vi "HeaderAction.vi"(0 "GenData en entrée":refnum<class "Tools.lvclass"> caption="DNL_LabVIEW Object in", 11 "error in (no error)":errorcluster caption="entrée d'erreur (pas d'erreur)") -> (4 "GenData en sortie":refnum<class "Tools.lvclass"> caption="DNL_LabVIEW Object out", 6 "DataNames":string[](array[string]), 8 "Instr Name":string, 10 "HeaderString":string, 13 "ArrDisplayNames":string[](array[string]), 14 "DisplayNames":string[](array[string]), 15 "error out":errorcluster caption="sortie d'erreur")   [LabVIEW 2019, in "Tools.lvclass"]
uses:
  Tools.lvclass
  C:/Programmes Labview/LabScanV1A/DevicesClass/BaseDevice/BaseDevice.lvclass
  Tools.lvclass/Tools.ctl
  BaseDevice/BaseDevice.lvclass
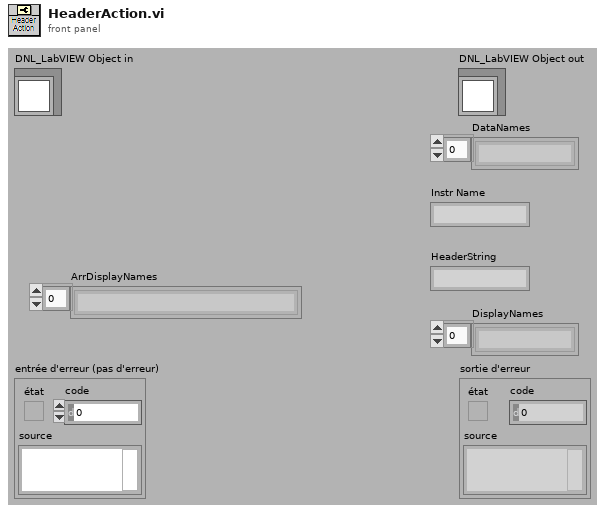
[diagram p1: front panel]
types:
  T1 = typedef "Tools.lvclass/Tools_Func.ctl" = enum16{"Courbe 1 (Arb)", "Courbe 2 (Arb)", "Courbe 3 (Arb)", "Courbe 123 (Arb,Arb,Arb)", "Scan Pos (Arb)", "Indice de Point (Points)", "AbsTime (ms)", "Minuteur (s)", "Panneaux Infos (Na)", "Délais (ms)", "RandwithDbind(Arb)", "RandomNum (Arb)", "Multisweep (Sw)", "ScanTime (s)"}
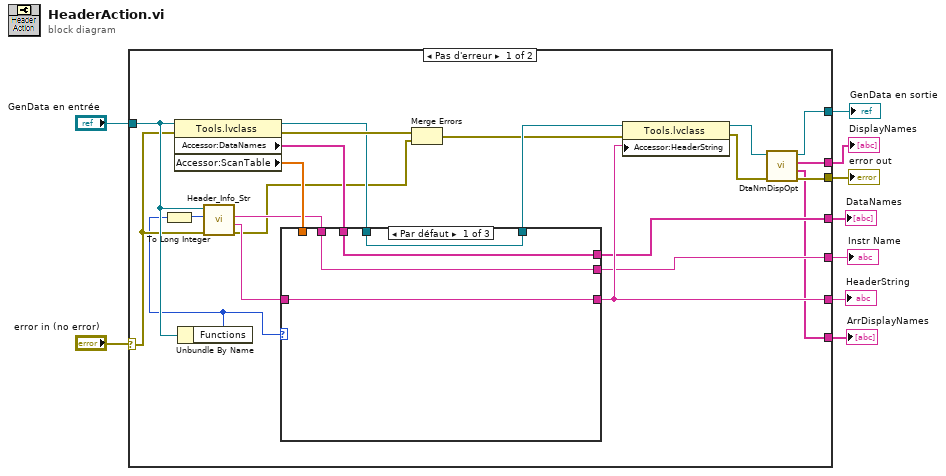
[diagram p0: block diagram]
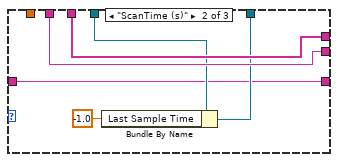
[diagram p2: hidden frame]
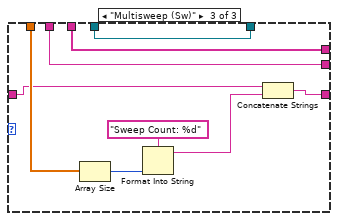
[diagram p3: hidden frame]
diagram:
  n1 = case shown="Pas d'erreur" "error in (no error)" {
    selector: "error in (no error)" -> [w17 w51]
    tunnel: [w30 _] -> w8
    tunnel: [w26 _] -> w7
    tunnel: "GenData en entrée" -> [w18 w52]
    tunnel: [w25 w51] -> w5
    tunnel: [w22 w52] -> w4
    tunnel: [w28 _] -> w3
    tunnel: [w21 _] -> w2
    tunnel: [w10 _] -> w1
    frame No Error {
      n2 = property class="Tools.lvclass"(reference=w18, error in=w17) -> (reference out=w20:refnum<class "Tools.lvclass">, error out=w31:errorcluster, "Accessor:DataNames"=w27:string[], "Accessor:ScanTable"=w29:dbl[])
      n3 = Unbundle By Name(w18) -> ("Functions"=w12:T1)
      n4 = To Long Integer(number=w12) -> (32bit integer=w11:i32)
      n5 = call-dynamic "Header_Info_Str.vi"("error in (no error)"=w17, "Functions"=w11, "DefaultDev in"=w18) -> ("error out"=w13:errorcluster, "HdrInfoStr"=w16:string, "InstrumentName"=w15:string)  [unwired: 5 in, 1 out]
      n6 = case shown="Par défaut" w12 {
        tunnel: [w32 w36 w43] -> w30
        tunnel: w29 -> [_ _ w50]
        tunnel: [w35 w40 w46] -> w28
        tunnel: w15 -> [w35 w40 w46]
        tunnel: w27 -> [w34 w41 w47]
        tunnel: [w34 w41 w47] -> w26
        tunnel: w20 -> [w33 w39 w44]
        tunnel: [w33 w38 w44] -> w19
        tunnel: w16 -> [w32 w36 w42]
        frame Default {
        }
        frame "ScanTime (s)" {
          n7 = Bundle By Name(cluster=w39, "Last Sample Time"=-1.0) -> (w38:refnum<class "Tools.lvclass">)
        }
        frame "Multisweep (Sw)" {
          n8 = Array Size(array=w50) -> (size(s)=w49:i32)
          n9 = Format Into String(format string="Sweep Count: %d" ("chaîne de format"), w49) -> (resulting string=w45:string)  [unwired: 2 in, 1 out]
          n10 = Concatenate Strings(w42, w45) -> (w43:string)
        }
      }
      n11 = Merge Errors(w31, w13) -> (w14:errorcluster)
      n12 = property class="Tools.lvclass"(reference=w19, error in=w14, "Accessor:HeaderString"=w30) -> (reference out=w23:refnum<class "Tools.lvclass">, error out=w24:errorcluster)
      n13 = call "DtaNmDispOpt.vi"("error in (no error)"=w24, "BaseDevice en entrée"=w23) -> ("error out"=w25:errorcluster, "ArrDisplayNames"=w10:string[], "DisplayNames"=w21:string[], "BaseDevice en sortie"=w22:refnum<class "Tools.lvclass">)  [unwired: 6 in]
    }
    frame Error {
    }
  }
  "error out" <- w5
  "GenData en sortie" <- w4
  "DataNames" <- w7
  "HeaderString" <- w8
  "Instr Name" <- w3
  "DisplayNames" <- w2
  "ArrDisplayNames" <- w1
